vi "Set Enable State on Multiple Controls.vi"(10 "Enable?":bool, 11 "Controls":refnum<vi>[](array[refnum])) -> ()   [LabVIEW 2017, in "CML UI.lvlib"]
doc: "Sets all the controls in the input array to the \"Enable state\" value.\n_____\nBased on Delacor QMH Project Template 4.1.0.56."
uses:
  CML UI.lvlib
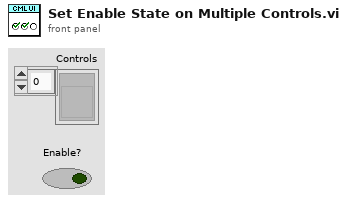
[diagram p1: front panel]
types:
  T1 = enum8{"Enabled", "Disabled", "Disabled and Grayed Out"}
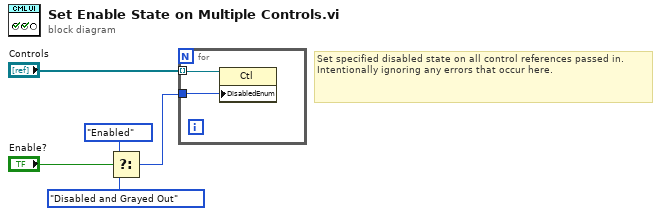
[diagram p0: block diagram]
diagram:
  # "Set specified disabled state on all control references passed in. Intentionally ignoring any errors that occur here."
  n1 = Select(t=T1."Enabled" ("Disabled"), s="Enable?", f=T1."Disabled and Grayed Out" ("Disabled")) -> (s? t:f=w3:T1)
  n2 = for {
    tunnel: "Controls" -> [w7] mode=indexing
    tunnel: w3 -> [w6]
    n3 = property on="Property Node" class="Ctl"(reference=w7, "DisabledEnum"=w6) -> ()  [unwired: 1 in, 2 out]
  }
